vi "Hood Limelight Jog.vi"(11 "Jog Amount":dbl) -> ()   [LabVIEW 2019]
doc: "This template is useful for immediate subsystem actions that do not need deadband filtering\n\nBe sure to right-click and select New from Template and save with a new command name."
uses:
  Turret/SynchronousVIs/LL Offsets.vi
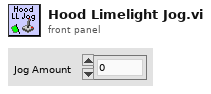
[diagram p1: front panel]
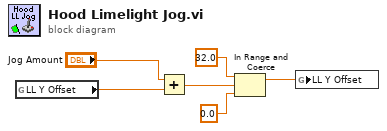
[diagram p0: block diagram]
diagram:
  n1 = global read "LL Offsets.vi" "LL Y Offset"() -> (w6:dbl)
  n2 = Add(x="Jog Amount", y=w6) -> (x+y=w4:dbl)
  n3 = In Range and Coerce(upper limit=32.0, x=w4, lower limit=0.0) -> (coerced(x)=w3:dbl)  [unwired: 1 out]
  n4 = global write "LL Offsets.vi" "LL Y Offset"(w3) -> ()
